vi "Main_WAV_Reader.vi"() -> ()   [LabVIEW 2022 SP3]
uses:
  PreferencesControl.ctl
  <vilib>/Waveform/WDTOps.llb/WDT Get Waveform Subset DBL.vi
panel:
  in  "Tab Control":enum32{"Instructions", "Settings"}(tab)
  out "Subplot":waveform(dbl)[](graph)
  in  "Default settings":T1={"Name of test"="WAV import", "Date"=timestamp(0 s since 1904-01-01), "Location"="Home", "Template"="None", "Soundcard"="Unknown", "resolution"=32, "Sampling rate"=48000, "Ch1 Gain "=0.0, "Ch2 Gain"=0.0, "Sample time (s)"=0.3, "Pre-trigger (s)"=0.001, "Hammer Threshold"=0.2, "Positions"=12, "Taps/Position"=4, "Set Names"="H", "Freq resolution"=1.0, "Hammer cutoff"=0.0015, "Mic cutoff"=0.3, "Double bounce "=0.1, "Hammer Cal"=1000.0, "dB Offset"=0.0, "Accel Cal"=1.0, "Vibrometer Cal"=1.0, "Mic Cal"=1000.0, "Output"=2, "Voltage Cal"=1.0, "Vibrometer Port"="ASRL27::INSTR", "Range"=1, "High Pass"=2, "Bandwidth"=1, "X Range"=[], "Y Range"=[], "dB Spread"=0.0, "Trigger"=0, "Ch_1"=1, "Ch_2"=2, "flip?"=FALSE, "60Hz"=FALSE, "Time offset"=0.0, "Piezo Cal"=1.0, "Default Notes"=""} {"Ch_2" min=1 step=1; "Ch_1" min=1 max=100 step=1; "Trigger" items=["Hammer (force)", "Self-tap", "Spacebar"]; "Bandwidth" items=["1 kHz"=1, "5 kHz"=5, "10 kHz"=10, "25 kHz"=25, "50 kHz"=50, "100 kHz"=100]; "High Pass" items=["Off", "13 Hz", "104 Hz"]; "Range" items=["10 mm/s"=1, "20 mm/s"=2, "50 mm/s"=5, "100 mm/s"=10, "200 mm/s"=20, "500 mm/s"=50, "1 m/s"=100, "2 m/s"=200]; "Output" items=["Accelerometer", "Speed (from acceleration)", "Microphone", "Vibrometer", "Piezo"]; "Voltage Cal" format="%#_13g"; "Ch2 Gain" format="%#_13g"; "Ch1 Gain" format="%#_13g"; "Double bounce" min=0.0; "Mic cutoff" min=0.0 format="%#_4g"; "Hammer cutoff" min=0.0 format="%#_4g"; "Freq resolution" min=0.0; "Pre-trigger (s)" format="%#_13g"; "Date" format="%<%H:%M\n%d/%m/%y>T"; "resolution" items=["16 bit"=16, "24 bit"=24, "32 bit"=32]; "Sampling rate" items=["22050 samp/s"=22050, "44100 samp/s"=44100, "48000 samp/s"=48000]}
  in  "Flag":bool
  out "Alarms":string
  in  "Save":bool
  out "sampling rate":dbl
  in  "path":path
  out "Average FRF":cluster{dbl, "df":dbl, dbl[]}[](graph)
  in  "View":u16(ring) items=["Raw", "Volts", "Units (Pa, N, etc)"]
  out "Hammer Spectrum":cluster{dbl, "df":dbl, "FFT {X}":dbl[]}[](graph)
  out "Hammer Data":cluster{dbl, "dt":dbl, "Y":dbl[]}[](graph)
  out "Microphone Data":cluster{dbl, "dt":dbl, "Y":dbl[]}[](graph)
  in  "Play":bool
  in  "reset":bool
  out "Array":cluster{"data":waveform(dbl)[]}[](array[cluster])
  in  "Params":T2={"Duration (s)"=0.3, "offset (s)"=0.001, "Threshold"=0.2763157894736842, "Positions"=12, "Taps/Position"=4, "Set Type"="H", "freq res"=1.0} {"Threshold" scale=0.0..1.0}
  out "# hits":dbl
  in  "First Channel":u16(ring)=1 items=["Hammer", "Microphone"]
  out "Complete Data Set":waveform(dbl)[](graph)
  # "Instructions:\n1. select your file\n2. adjust both yellow cursors \n     to select the subset you want to save\n3. adjust the purple threshold line on the \n     hammer plot if you need to\n4. make sure you have the output channel\n     in red (otherwise change the \"First\n     Channel\" selection)\n5. Hit Export to save and select an \n     instrument and test name"
  # "Hz"
  # "dB"
  # "dB"
  # "sec"
  # "sec"
  # "mV/Pa"
  # "mV/m/s2"
  # "mV/mm/s"
  # "V/N"
  # "sec"
  # "sec"
  # "mV/N"
  # "a.u."
  # "a.u."
  # "sec"
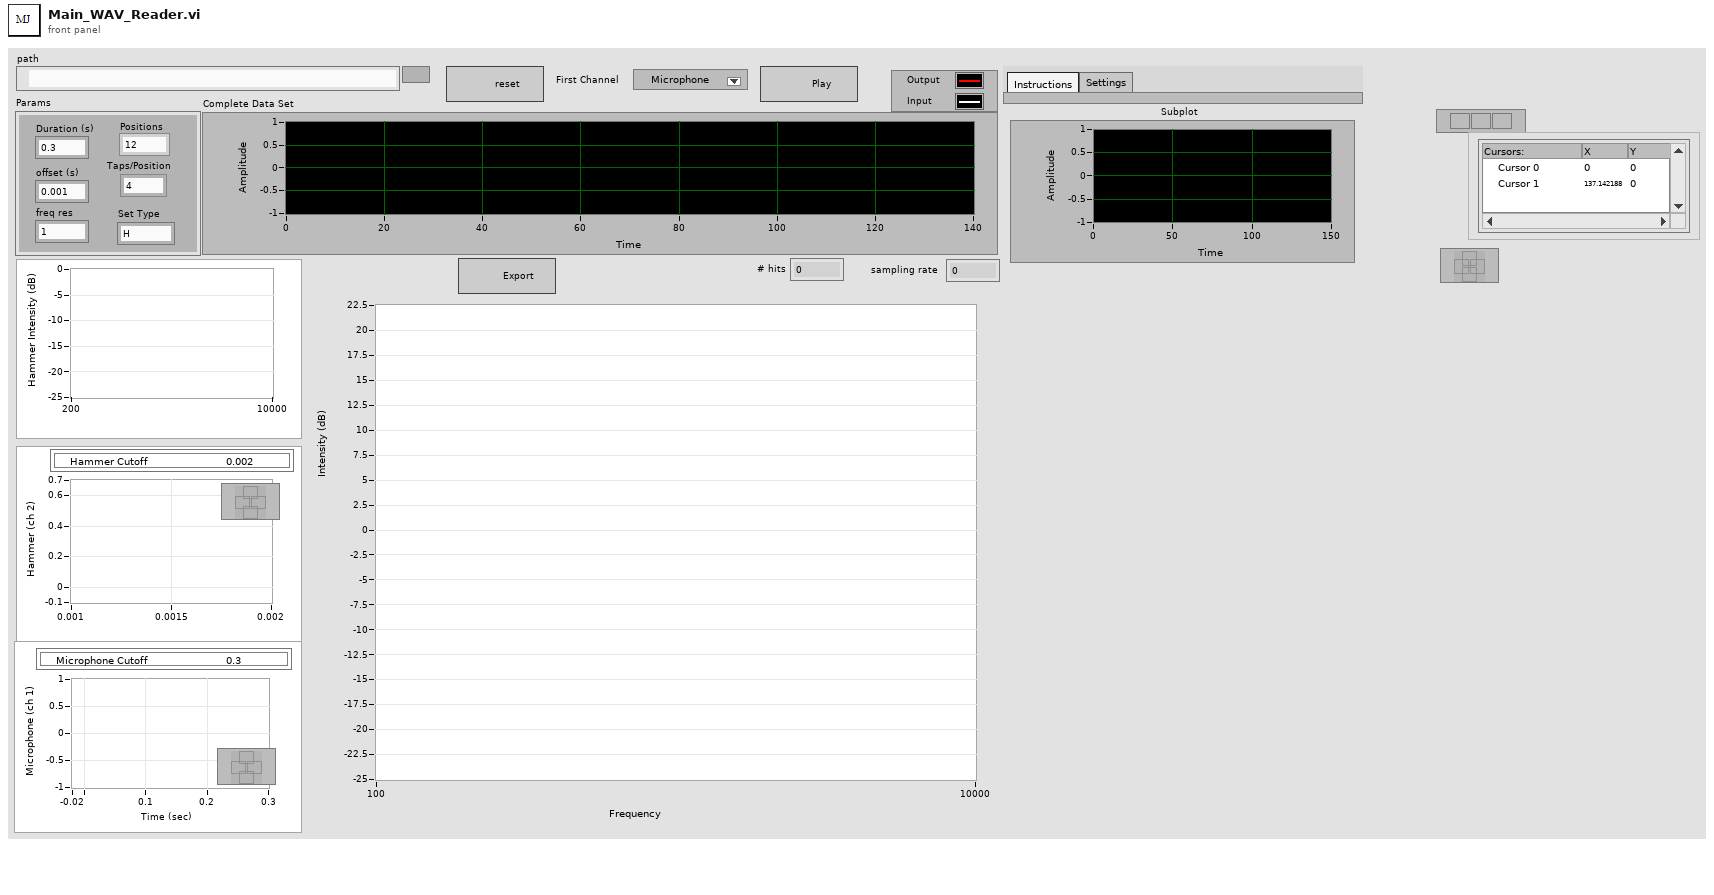
[diagram p1: front panel]
types:
  T1 = typedef "PreferencesControl.ctl" = cluster{"Name of test":string, "Date":timestamp, "Location":string, "Template":string, "Soundcard":string, "resolution":u16, "Sampling rate":u16, "Ch1 Gain ":dbl, "Ch2 Gain":dbl, "Sample time (s)":dbl, "Pre-trigger (s)":dbl, "Hammer Threshold":dbl, "Positions":i16, "Taps/Position":i16, "Set Names":string, "Freq resolution":dbl, "Hammer cutoff":dbl, "Mic cutoff":dbl, "Double bounce ":dbl, "Hammer Cal":dbl, "dB Offset":dbl, "Accel Cal":dbl, "Vibrometer Cal":dbl, "Mic Cal":dbl, "Output":u16, "Voltage Cal":dbl, "Vibrometer Port":refnum<visa-resource-name>, "Range":u16, "High Pass":u16, "Bandwidth":u16, "X Range":cluster{"Minimum":dbl, "Maximum":dbl, "Increment":dbl, "Minor Increment":dbl, "Start":dbl}[], "Y Range":cluster{"Minimum":dbl, "Maximum":dbl, "Increment":dbl, "Minor Increment":dbl, "Start":dbl}[], "dB Spread":dbl, "Trigger":u16, "Ch_1":u8, "Ch_2":u8, "flip?":bool, "60Hz":bool, "Time offset":dbl, "Piezo Cal":dbl, "Default Notes":string}
  T2 = cluster{"Duration (s)":dbl, "offset (s)":dbl, "Threshold":dbl, "Positions":i16, "Taps/Position":i16, "Set Type":string, "freq res":dbl}
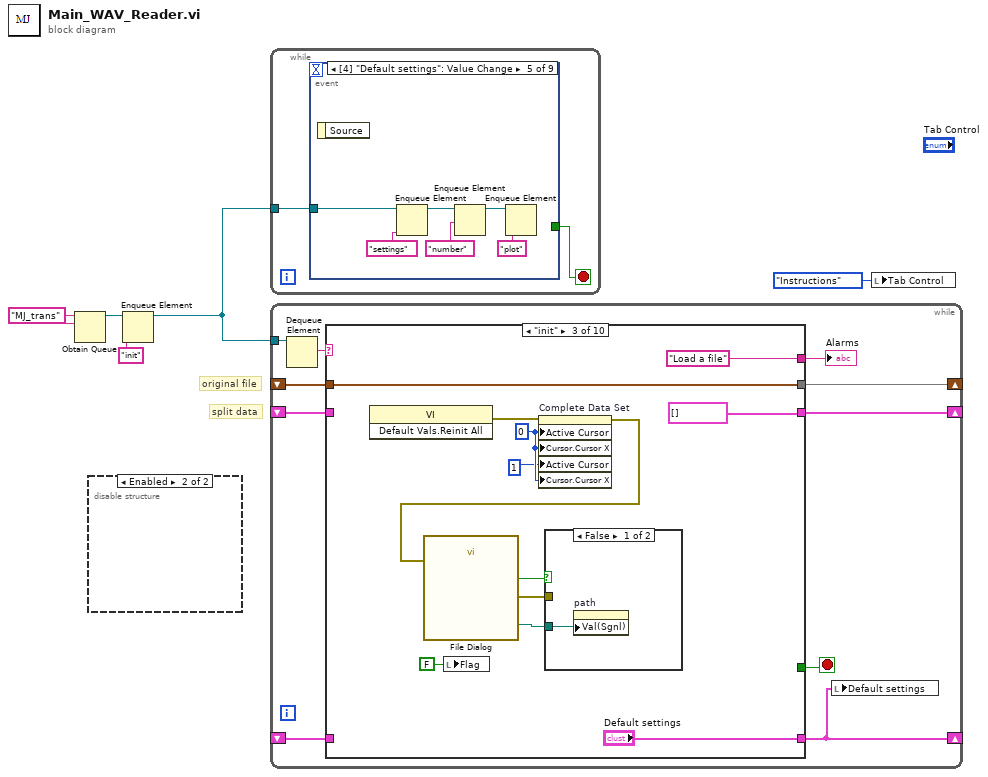
[diagram p0: block diagram]
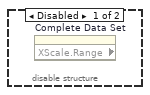
[diagram p2: hidden frame]
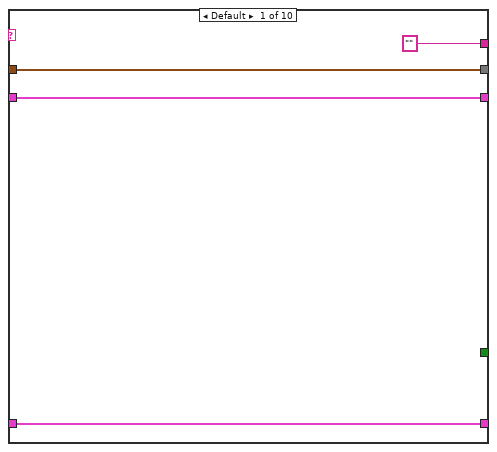
[diagram p3: hidden frame]
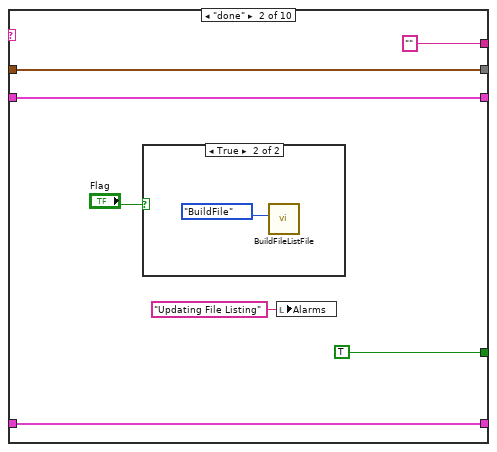
[diagram p4: hidden frame]
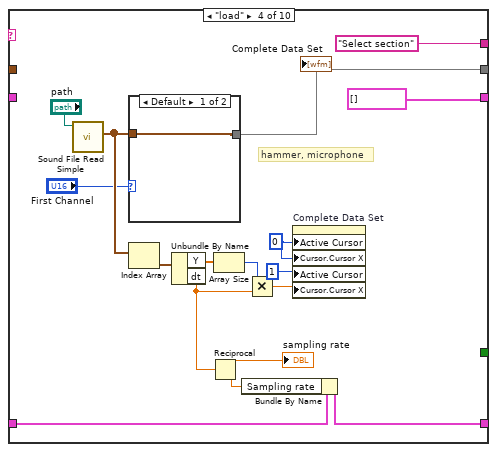
[diagram p7: hidden frame]
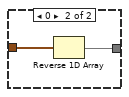
[diagram p8: hidden frame]
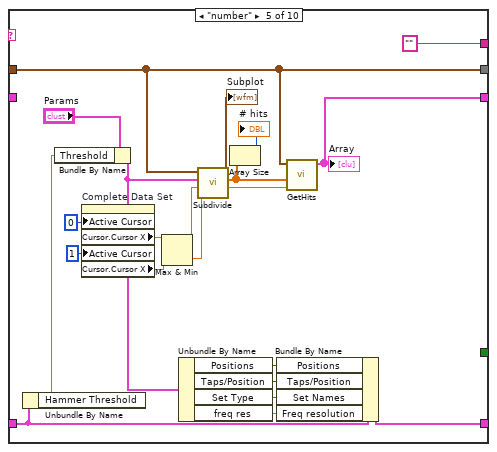
[diagram p9: hidden frame]
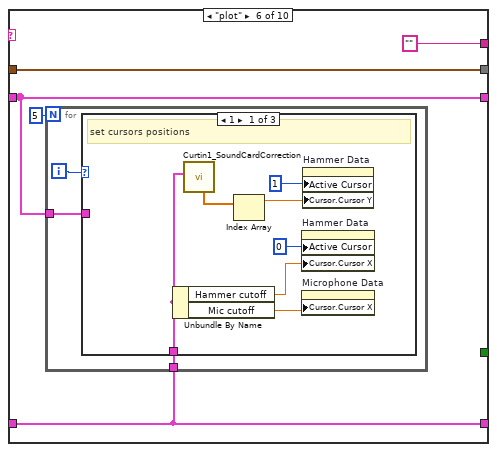
[diagram p10: hidden frame]
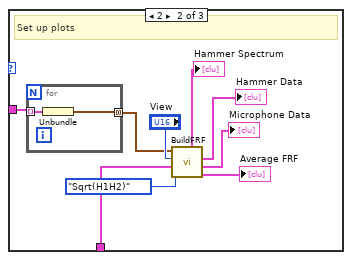
[diagram p11: hidden frame]
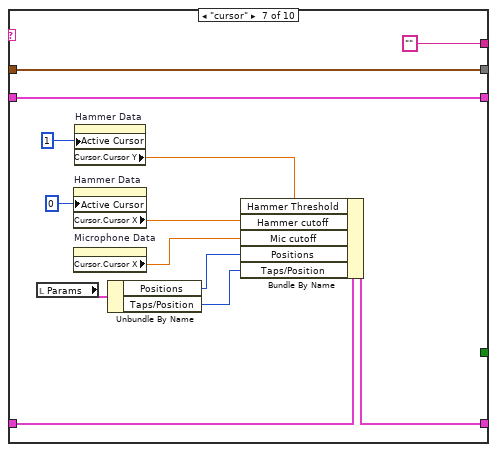
[diagram p13: hidden frame]
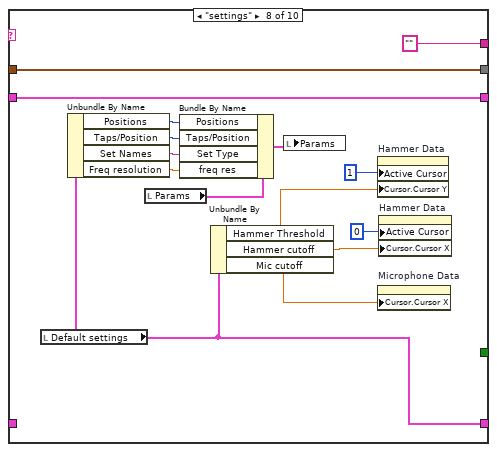
[diagram p14: hidden frame]
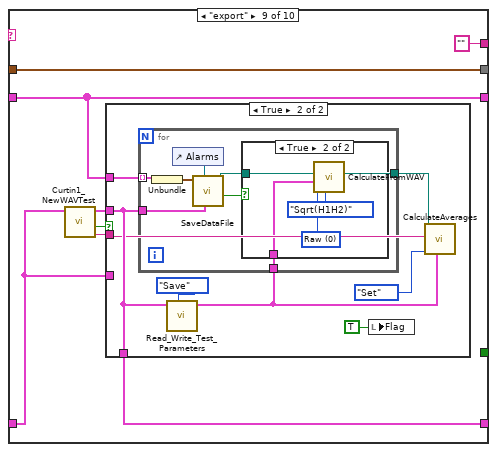
[diagram p15: hidden frame]
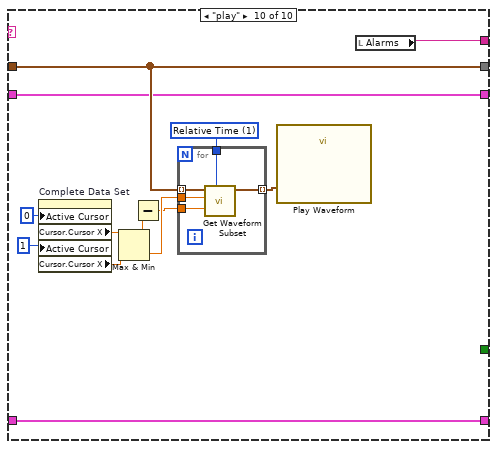
[diagram p18: hidden frame]
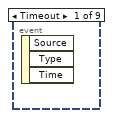
[diagram p19: hidden frame]
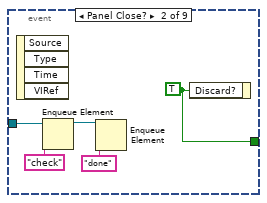
[diagram p20: hidden frame]
diagram:
  w4 = "MJ_trans" ("name (unnamed)")
  # "split data"
  # "original file"
  n1 = Obtain Queue(name (unnamed)=w4, element data type=w4) -> (queue out=w5:refnum<queue>)  [unwired: 3 in, 2 out]
  n2 = disable-structure shown="Enabled" {
    frame Disabled {
      n3 = property on="Complete Data Set" class="WFGraph (strict)" props=["XScale", "Range"]() -> ()  [unwired: 2 in, 3 out]
    }
    frame Enabled {
    }
  }
  n4 = Enqueue Element(queue=w5, element="init") -> (queue out=w2:refnum<queue>)  [unwired: 2 in, 2 out]
  n5 = while {
    tunnel: w2 -> [w6]
    stop <- w7 stop-if-true
    n6 = event shown="[4] \"Default settings\": Value Change" {
      selector: _ -> [_ _ _ _ _ _ _ _ _]
      dyn-events: _ -> [_ _ _ _ _ _ _ _ _]
      timeout: _ -> [_ _ _ _ _ _ _ _ _]
      tunnel: [_ w12 _ _ _ _ _ _ _] -> w7
      tunnel: w6 -> [_ w9 w15 w17 w23 w25 w31 w33 w39]
      event Timeout {
        n7 = event-data() -> ()  [unwired: 1 in, 3 out]
      }
      event Panel Close? {
        w12 = TRUE ("Discard?")
        n8 = event-data() -> ()  [unwired: 1 in, 4 out]
        n9 = Enqueue Element(queue=w9, element="check") -> (queue out=w8:refnum<queue>)  [unwired: 2 in, 2 out]
        n10 = Enqueue Element(queue=w8, element="done") -> ()  [unwired: 2 in, 3 out]
        n11 = event-data("Discard?"=w12) -> ()  [unwired: 1 in, 1 out]
      }
      event "Complete Data Set": Cursor Release {
        n12 = event-data() -> ()  [unwired: 1 in, 1 out]
        n13 = Enqueue Element(queue=w15, element="number") -> (queue out=w13:refnum<queue>)  [unwired: 2 in, 2 out]
        n14 = Enqueue Element(queue=w13, element="plot") -> ()  [unwired: 2 in, 3 out]
      }
      event "reset": Value Change {
        n15 = event-data() -> ()  [unwired: 1 in, 1 out]
        n16 = Enqueue Element(queue=w17, element="load") -> ()  [unwired: 2 in, 3 out]
      }
      event Value Change {
        n17 = event-data() -> ()  [unwired: 1 in, 1 out]
        n18 = Enqueue Element(queue=w23, element="settings") -> (queue out=w19:refnum<queue>)  [unwired: 2 in, 2 out]
        n19 = Enqueue Element(queue=w19, element="number") -> (queue out=w20:refnum<queue>)  [unwired: 2 in, 2 out]
        n20 = Enqueue Element(queue=w20, element="plot") -> ()  [unwired: 2 in, 3 out]
      }
      event "Play": Value Change {
        n21 = event-data() -> ()  [unwired: 1 in, 1 out]
        n22 = Enqueue Element(queue=w25, element="play") -> ()  [unwired: 2 in, 3 out]
      }
      event "path": Value Change {
        n23 = event-data() -> ()  [unwired: 1 in, 1 out]
        n24 = Enqueue Element(queue=w31, element="load") -> (queue out=w29:refnum<queue>)  [unwired: 2 in, 2 out]
        n25 = Enqueue Element(queue=w29, element="number") -> (queue out=w27:refnum<queue>)  [unwired: 2 in, 2 out]
        n26 = Enqueue Element(queue=w27, element="plot") -> ()  [unwired: 2 in, 3 out]
      }
      event "Save": Value Change {
        n27 = event-data() -> ()  [unwired: 1 in, 3 out]
        n28 = Enqueue Element(queue=w33, element="export") -> ()  [unwired: 2 in, 3 out]
      }
      event "Hammer Spectrum", "Hammer Data", "Microphone Data": Cursor Release; "First Channel", "Params": Value Change {
        n29 = event-data() -> ()  [unwired: 1 in, 4 out]
        n30 = Enqueue Element(queue=w39, element="cursor") -> (queue out=w37:refnum<queue>)  [unwired: 2 in, 2 out]
        n31 = Enqueue Element(queue=w37, element="number") -> (queue out=w35:refnum<queue>)  [unwired: 2 in, 2 out]
        n32 = Enqueue Element(queue=w35, element="plot") -> ()  [unwired: 2 in, 3 out]
      }
    }
  }
  n33 = while {
    tunnel: w2 -> [w50]
    shift-right: [w47] -> _
    shift-left: _ -> [w46]
    shift-right: [w45] -> _
    shift-left: _ -> [w44]
    shift-right: [w41] -> _
    shift-left: _ -> [w42]
    stop <- w48 stop-if-true
    n34 = Dequeue Element(queue=w50) -> (element=w49:string)  [unwired: 2 in, 3 out]
    n35 = case shown="\"init\"" w49 {
      tunnel: [_ TRUE _ _ _ _ _ _ _ _] -> w48
      tunnel: [w54 w60 w74 w90 w109 w120 w155 w170 w178 w207] -> w47
      tunnel: w46 -> [w54 w60 w74 _ w109 w120 w155 w170 w178 w207]
      tunnel: [w53 w59 cluster{waveform(dbl)[]}[] [] ("Array out") cluster{waveform(dbl)[]}[] [] ("Array out") w106 w119 w154 w169 w176 w201] -> w45
      tunnel: w44 -> [w53 w59 _ _ _ w119 w154 w169 w176 w201]
      tunnel: ["" ("Alarms") "" ("Alarms") "Load a file" ("Alarms") "Select section" ("Alarms") "" ("Alarms") "" ("Alarms") "" ("Alarms") "" ("Alarms") "" ("Alarms") w200] -> w43
      tunnel: w42 -> [w51 w57 _ w77 w102 w117 w147 _ w172 w199]
      tunnel: [w51 w57 "Default settings" w76 w96 w117 w146 w159 w173 w199] -> w41
      frame Default {
      }
      frame "done" {
        n36 = case shown="True" "Flag" {
          frame False {
          }
          frame True {
            n37 = call "BuildFileListFile.vi"("Task"=enum16{"BuildFile", "ReadFile"}."BuildFile") -> ()  [unwired: 9 in, 2 out]
          }
        }
        n38 = local write "Alarms"("Updating File Listing" ("Alarms")) -> ()
      }
      frame "init" {
        w73 = 0 ("Cursor.Cursor Index")
        n39 = invoke class="VI" method="Default Vals.Reinit All"() -> (error out=w65:errorcluster)  [unwired: 3 in, 2 out]
        n40 = local write "Flag"(FALSE ("Flag")) -> ()
        n41 = property on="Complete Data Set" class="WFGraph (strict)"(error in=w65, "Active Cursor"=w73, "Cursor.Cursor X"=w73, "Active Cursor"=1 ("Cursor.Cursor Index"), "Cursor.Cursor X"=w73) -> (error out=w66:errorcluster)  [unwired: 1 in, 1 out]
        n42 = call "File Dialog"("error in"=w66) -> ("selected path"=w72:path, "cancelled"=w71:bool, "error out"=w69:errorcluster)  [unwired: 11 in, 1 out]
        n43 = case shown="False" w71 {
          tunnel: w72 -> [w75 _]
          tunnel: w69 -> [_ _]
          frame False {
            n44 = property on="path" class="Path"("Val(Sgnl)"=w75) -> ()  [unwired: 2 in, 2 out]
          }
          frame True {
          }
        }
      }
      frame "load" {
        w85 = 0 ("Cursor.Cursor Index")
        # "hammer, microphone"
        n45 = call <vilib>:"Sound File Read Simple.vi"("path"="path") -> ("data"=w89:waveform(dbl)[])  [unwired: 7 in, 3 out]
        n46 = case shown="Default" "First Channel" {
          tunnel: w89 -> [w92 w94]
          tunnel: [w92 w93] -> w90
          frame Default {
          }
          frame 0 {
            n47 = Reverse 1D Array(array=w94) -> (reversed array=w93:waveform(dbl)[])
          }
        }
        "Complete Data Set" <- w90
        n48 = Index Array(array=w89) -> (element=w88:waveform(dbl))  [unwired: 1 in]
        n49 = Unbundle By Name(w88) -> ("Y"=w87:dbl[], "dt"=w82:dbl)
        n50 = Reciprocal(x=w82) -> (1/x=w81:dbl)
        "sampling rate" <- w81
        n51 = Array Size(array=w87) -> (size(s)=w84:i32)
        n52 = Bundle By Name(cluster=w77, "Sampling rate"=w81) -> (w76:T1)
        n53 = Multiply(x=w84, y=w82) -> (x*y=w83:dbl)
        n54 = property on="Complete Data Set" class="WFGraph (strict)"("Active Cursor"=w85, "Cursor.Cursor X"=w85, "Active Cursor"=1 ("Cursor.Cursor Index"), "Cursor.Cursor X"=w83) -> ()  [unwired: 2 in, 2 out]
      }
      frame "number" {
        n55 = Unbundle By Name(w102) -> ("Hammer Threshold"=w103:dbl)
        n56 = Bundle By Name(cluster="Params", "Threshold"=w103) -> (w101:T2)
        n57 = property on="Complete Data Set" class="WFGraph (strict)"("Active Cursor"=0 ("Cursor.Cursor Index"), "Active Cursor"=1 ("Cursor.Cursor Index")) -> ("Cursor.Cursor X"=w114:dbl, "Cursor.Cursor X"=w113:dbl)  [unwired: 2 in, 2 out]
        n58 = Max & Min(x=w114, y=w113) -> (max(x,y)=w112:dbl, min(x,y)=w111:dbl)
        n59 = Unbundle By Name(w101) -> ("Positions"=w100:i16, "Taps/Position"=w99:i16, "Set Type"=w97:string, "freq res"=w95:dbl)
        n60 = call "Subdivide.vi"("Minimum"=w111, "Maximum"=w112, "Params"=w101, "Waveform Graph"=w109) -> ("duration (pts)"=w108:dbl, "Array"=w107:dbl[], "Waveform Graph 2"=→"Subplot":waveform(dbl)[])  [unwired: 5 in]
        n61 = Array Size(array=w107) -> (size(s)=→"# hits":i32)
        n62 = Bundle By Name(cluster=w102, "Positions"=w100, "Taps/Position"=w99, "Set Names"=w97, "Freq resolution"=w95) -> (w96:T1)
        n63 = call "GetHits.vi"("duration (pts)"=w108, "Array in"=w107, "data"=w109) -> ("Array"=w106:cluster{"data":waveform(dbl)[]}[])  [unwired: 8 in]
        "Array" <- w106
      }
      frame "plot" {
        n64 = for {
          N: 5 ("timeout in ms (-1)") -> [_]
          tunnel: w117 -> [w123]
          tunnel: w119 -> [w122]
          i -> [w124]
          n65 = case shown="1" w124 {
            tunnel: w123 -> [w127 w138 _]
            tunnel: w122 -> [_ w132 _]
            frame 1 {
              # "set cursors positions"
              n66 = Unbundle By Name(w127) -> ("Hammer cutoff"=w131:dbl, "Mic cutoff"=w130:dbl)
              n67 = call "Curtin1_SoundCardCorrection.vi"("Settings"=w127) -> ("Converted"=w126:dbl[])  [unwired: 5 in, 5 out]
              n68 = Index Array(array=w126) -> (element=w125:dbl)  [unwired: 1 in]
              n69 = property on="Hammer Data" class="WFGraph (strict)"("Active Cursor"=u32 0, "Cursor.Cursor X"=w131) -> ()  [unwired: 2 in, 2 out]
              n70 = property on="Microphone Data" class="WFGraph (strict)"("Cursor.Cursor X"=w130) -> ()  [unwired: 2 in, 2 out]
              n71 = property on="Hammer Data" class="WFGraph (strict)"("Active Cursor"=u32 1, "Cursor.Cursor Y"=w125) -> ()  [unwired: 2 in, 2 out]
            }
            frame 2 {
              # "Set up plots"
              n72 = for {
                tunnel: w132 -> [w142] mode=indexing
                tunnel: [w141] -> w134 mode=concatenating
                n73 = Unbundle(w142) -> ("data"=w141:waveform(dbl)[])
              }
              n74 = call "BuildFRF.vi"("Method"=enum16{"Sqrt(H1H2)", "H1", "H2"}."Sqrt(H1H2)", "Settings"=w138, "View"="View", "Data In"=w134) -> ("Average FRF"=→"Average FRF":cluster{dbl, "df":dbl, dbl[]}[], "Microphone"=→"Microphone Data":cluster{dbl, "dt":dbl, "Y":dbl[]}[], "Hammer"=→"Hammer Data":cluster{dbl, "dt":dbl, "Y":dbl[]}[], "Hammer Spectra"=→"Hammer Spectrum":cluster{dbl, "df":dbl, "FFT {X}":dbl[]}[])  [unwired: 2 in, 2 out]
            }
            frame Default {
            }
          }
        }
      }
      frame "cursor" {
        n75 = local read "Params"() -> (w145:T2)
        n76 = property on="Hammer Data" class="WFGraph (strict)"("Active Cursor"=u32 0) -> ("Cursor.Cursor X"=w149:dbl)  [unwired: 2 in, 2 out]
        n77 = property on="Microphone Data" class="WFGraph (strict)"() -> ("Cursor.Cursor X"=w148:dbl)  [unwired: 2 in, 2 out]
        n78 = property on="Hammer Data" class="WFGraph (strict)"("Active Cursor"=u32 1) -> ("Cursor.Cursor Y"=w150:dbl)  [unwired: 2 in, 2 out]
        n79 = Unbundle By Name(w145) -> ("Positions"=w144:i16, "Taps/Position"=w143:i16)
        n80 = Bundle By Name(cluster=w147, "Hammer Threshold"=w150, "Hammer cutoff"=w149, "Mic cutoff"=w148, "Positions"=w144, "Taps/Position"=w143) -> (w146:T1)
      }
      frame "settings" {
        n81 = local read "Default settings"() -> (w159:T1)
        n82 = Unbundle By Name(w159) -> ("Positions"=w160:i16, "Taps/Position"=w161:i16, "Set Names"=w162:string, "Freq resolution"=w156:dbl)
        n83 = local read "Params"() -> (w158:T2)
        n84 = Bundle By Name(cluster=w158, "Positions"=w160, "Taps/Position"=w161, "Set Type"=w162, "freq res"=w156) -> (w157:T2)
        n85 = Unbundle By Name(w159) -> ("Hammer Threshold"=w165:dbl, "Hammer cutoff"=w164:dbl, "Mic cutoff"=w163:dbl)
        n86 = local write "Params"(w157) -> ()
        n87 = property on="Hammer Data" class="WFGraph (strict)"("Active Cursor"=u32 1, "Cursor.Cursor Y"=w165) -> ()  [unwired: 2 in, 2 out]
        n88 = property on="Microphone Data" class="WFGraph (strict)"("Cursor.Cursor X"=w163) -> ()  [unwired: 2 in, 2 out]
        n89 = property on="Hammer Data" class="WFGraph (strict)"("Active Cursor"=u32 0, "Cursor.Cursor X"=w164) -> ()  [unwired: 2 in, 2 out]
      }
      frame "export" {
        n90 = call "Curtin1_NewWAVTest.vi"("Settings"=w172) -> ("Instrument -- test out"=w171:string, "updated?"=w175:bool, "Settings out"=w174:T1)  [unwired: 8 in]
        n91 = case shown="True" w175 {
          tunnel: w176 -> [_ w187]
          tunnel: w174 -> [_ w185]
          tunnel: [w179 w185] -> w173
          tunnel: w172 -> [w179 _]
          tunnel: w171 -> [_ w181]
          frame False {
          }
          frame True {
            n92 = call "Read_Write_Test_Parameters.vi"("Task"=enum16{"Save", "Read", "Clear"}."Save", "Settings"=w185) -> ("Settings"=w180:T1)  [unwired: 8 in, 1 out]
            n93 = for {
              tunnel: w187 -> [w193] mode=indexing
              tunnel: w185 -> [w192]
              tunnel: w180 -> [w189]
              tunnel: [w188] -> w182
              n94 = Unbundle(w193) -> ("data"=w191:waveform(dbl)[])
              n95 = control-ref of="Alarms"() -> (w194:refnum<vi>)
              n96 = call "SaveDataFile.vi"("Settings"=w192, "Alarms"=w194, "Data"=w191) -> ("last tap?"=w190:bool, "new path"=w188:path)  [unwired: 4 in, 3 out]
              n97 = case shown="True" w190 {
                tunnel: w188 -> [_ w197]
                tunnel: w189 -> [_ w196]
                frame False {
                }
                frame True {
                  w195 = u16 0 items=["Raw", "Volts", "Units (Pa, N, etc)"] ("View")
                  n98 = call "CalculateFromWAV.vi"("Method"=enum16{"Sqrt(H1H2)", "H1", "H2"}."Sqrt(H1H2)", "View"=w195, "Settings"=w196, "path"=w197) -> ()  [unwired: 3 in, 5 out]
                }
              }
            }
            n99 = local write "Flag"(TRUE ("Flag")) -> ()
            n100 = call "CalculateAverages.vi"("Settings"=w180, "Task"=enum16{"Set", "Test"}."Set", "Inst:Test Name"=w181, "Last Data File"=w182) -> ()  [unwired: 8 in]
          }
        }
      }
      frame "play" {
        w203 = u16 1 items=["Samples", "Relative Time"] ("start/duration format")
        n101 = property on="Complete Data Set" class="WFGraph (strict)"("Active Cursor"=0 ("Cursor.Cursor Index"), "Active Cursor"=1 ("Cursor.Cursor Index")) -> ("Cursor.Cursor X"=w211:dbl, "Cursor.Cursor X"=w210:dbl)  [unwired: 2 in, 2 out]
        n102 = Max & Min(x=w211, y=w210) -> (max(x,y)=w206:dbl, min(x,y)=w205:dbl)
        n103 = Subtract(x=w206, y=w205) -> (x-y=w204:dbl)
        n104 = for {
          tunnel: w207 -> [w216] mode=indexing
          tunnel: w205 -> [w215]
          tunnel: w204 -> [w214]
          tunnel: w203 -> [w213]
          tunnel: [w212] -> w202 mode=indexing
          n105 = call-poly <vilib>:"Get Waveform Subset.vi"("start/duration format"=w213, "duration"=w214, "start samples/time"=w215, "waveform in"=w216) -> ("waveform out"=w212:waveform(dbl))  [unwired: 2 in, 3 out]
        }
        n106 = call "Play Waveform"("Data"=w202) -> ()  [unwired: 18 in, 1 out]
        n107 = local read "Alarms"() -> (w200:string)
      }
    }
    "Alarms" <- w43
    n108 = local write "Default settings"(w41) -> ()
  }
  n109 = local write "Tab Control"(enum32{"Instructions", "Settings"}."Instructions" ("Tab Control")) -> ()
